vi "PH_GUI.set I16 GUI object.vi"(2 "I16 GUI Ref":refnum<vi>, 3 "value":i16 caption="status", 4 "blinking (false)":bool, 5 "error in (no error)":errorcluster) -> (19 "error out":errorcluster)   [LabVIEW 2014, in "PH_Common.lvlib"]
doc: "Sets value and more for the referenced GUI object."
uses:
  PH_Common.lvlib
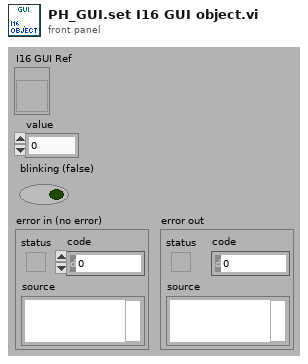
[diagram p1: front panel]
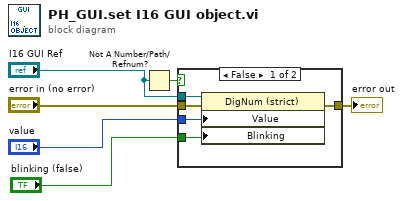
[diagram p0: block diagram]
diagram:
  n1 = Not A Number/Path/Refnum?(number/path/refnum="I16 GUI Ref") -> (NaN/Path/Refnum?=w3:bool)
  n2 = case shown="False" w3 {
    tunnel: "I16 GUI Ref" -> [w10 _]
    tunnel: "error in (no error)" -> [w11 w12]
    tunnel: [w9 w12] -> w5
    tunnel: "value" -> [w8 _]
    tunnel: "blinking (false)" -> [w7 _]
    frame False {
      n3 = property class="DigNum (strict)"(reference=w10, error in=w11, "Value"=w8, "Blinking"=w7) -> (error out=w9:errorcluster)  [unwired: 1 out]
    }
    frame True {
    }
  }
  "error out" <- w5
